vi "mod_PM CE Modulation.vi"(7 "carrier phase (rad)":dbl format="%.2f", 8 "kp":dbl format="%.4f", 11 "x":dbl[](array[numeric]) format="%.2f") -> (3 "PM CE":cdb[](array[numeric]) format="%.2f")   [LabVIEW 2020, in "niAMT.lvlib"]
doc: "This VI performs PM modulation of incoming message signal. The output is the base band complex envelope of PM signal."
uses:
  <vilib>/addons/Modulation/niAMT.lvlib
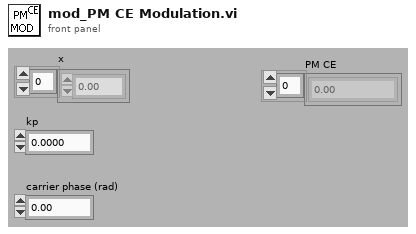
[diagram p1: front panel]
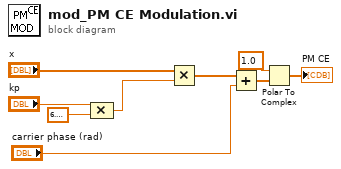
[diagram p0: block diagram]
diagram:
  n1 = Compound Arithmetic op=MULTIPLY("kp", 6.283185307179586) -> (w3:dbl)
  n2 = Multiply(x="x", y=w3) -> (x*y=w4:dbl[])
  n3 = Add(x=w4, y="carrier phase (rad)") -> (x+y=w2:dbl[])
  n4 = Polar To Complex(1:w2, 2:1.0) -> (0:→"PM CE":cdb[])
